vi "SubVI Caudal a Nivel peristaltica.vi"(11 "Numeric in":i32) -> (3 "Numeric out":dbl)   [LabVIEW 2013]
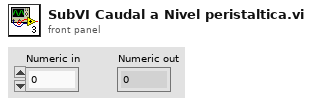
[diagram p1: front panel]
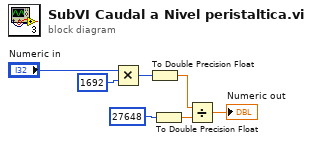
[diagram p0: block diagram]
diagram:
  n1 = Multiply(x="Numeric in", y=1692) -> (x*y=w4:i32)
  n2 = To Double Precision Float(number=w4) -> (double precision float=w2:dbl)
  n3 = To Double Precision Float(number=27648 ("y")) -> (double precision float=w1:dbl)
  n4 = Divide(x=w2, y=w1) -> (x/y=→"Numeric out":dbl)
